vi "VI Tree.vi"   [LabVIEW 2018, in "Agilent N6700 Series.lvlib"]
doc: "This is the instrument driver for the Keysight/Agilent N6700 Series.\nThe VI Tree displays all the user-callable VIs of the instrument driver in an organized table."
uses:
  Agilent N6700 Series.lvlib
  Configuration/Waveform/Configure Waveform (Exponential).vi
  Configuration/Waveform/Sequence/Configure Sequence (Exponential).vi
panel:
  # "(c) 2004-2019  National Instruments.  ALL RIGHTS RESERVED."
  # "SEE DIAGRAM\nFOR VI TREE."
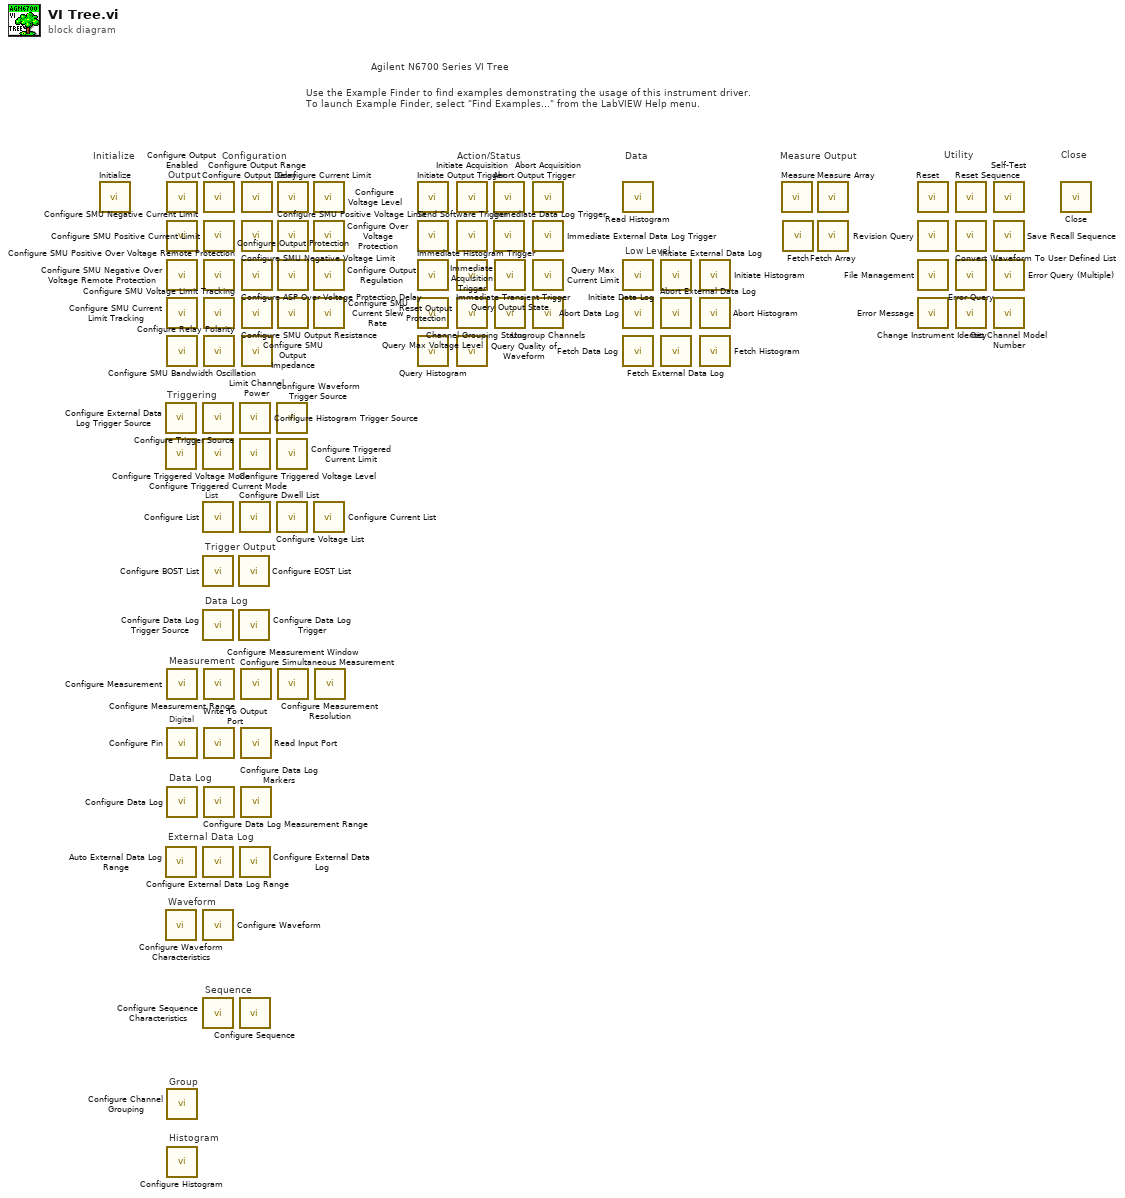
[diagram p0: block diagram]
diagram:
  # "External Data Log"
  # "Low Level"
  # "Sequence"
  # "Waveform"
  # "Data Log"
  # "Histogram"
  # "Data"
  # "Data Log"
  # "Measure Output"
  # "Agilent N6700 Series VI Tree"
  # "Use the Example Finder to find examples demonstrating the usage of this instrument driver.\nTo launch Example Finder, select \"Find Examples...\" from the LabVIEW Help menu."
  # "Configuration"
  # "Utility"
  # "Action/Status"
  # "Close"
  # "Initialize"
  # "Group"
  # "Digital"
  # "Measurement"
  # "Trigger Output"
  # "List"
  # "Triggering"
  # "Output"
  n1 = call "Initialize.vi"() -> ()  [unwired: 14 in, 2 out]
  n2 = call "Configure External Data Log Trigger Source.vi"() -> ()  [unwired: 10 in, 2 out]
  n3 = call "Configure Triggered Voltage Mode.vi"() -> ()  [unwired: 10 in, 2 out]
  n4 = call "Auto External Data Log Range.vi"() -> ()  [unwired: 10 in, 2 out]
  n5 = call "Configure Waveform Characteristics.vi"() -> ()  [unwired: 10 in, 2 out]
  n6 = call "Configure Output Enabled.vi"() -> ()  [unwired: 10 in, 2 out]
  n7 = call "Configure SMU Negative Current Limit.vi"() -> ()  [unwired: 10 in, 2 out]
  n8 = call "Configure SMU Negative Over Voltage Remote Protection.vi"() -> ()  [unwired: 10 in, 2 out]
  n9 = call "Configure SMU Current Limit Tracking.vi"() -> ()  [unwired: 10 in, 2 out]
  n10 = call "Configure SMU Bandwidth Oscillation.vi"() -> ()  [unwired: 10 in, 2 out]
  n11 = call "Configure Measurement.vi"() -> ()  [unwired: 10 in, 2 out]
  n12 = call "Configure Pin.vi"() -> ()  [unwired: 10 in, 2 out]
  n13 = call "Configure Data Log.vi"() -> ()  [unwired: 10 in, 2 out]
  n14 = call "Configure Channel Grouping.vi"() -> ()  [unwired: 10 in, 2 out]
  n15 = call "Configure Histogram.vi"() -> ()  [unwired: 10 in, 2 out]
  n16 = call "Configure Trigger Source.vi"() -> ()  [unwired: 10 in, 2 out]
  n17 = call "Configure Triggered Current Mode.vi"() -> ()  [unwired: 10 in, 2 out]
  n18 = call "Configure List.vi"() -> ()  [unwired: 10 in, 2 out]
  n19 = call "Configure BOST List.vi"() -> ()  [unwired: 10 in, 2 out]
  n20 = call "Configure Data Log Trigger Source.vi"() -> ()  [unwired: 10 in, 2 out]
  n21 = call "Configure External Data Log Range.vi"() -> ()  [unwired: 10 in, 2 out]
  n22 = call-poly "Configure Waveform.vi"() -> ()  [unwired: 14 in, 2 out]
  n23 = call "Configure Sequence Characteristics.vi"() -> ()  [unwired: 14 in, 2 out]
  n24 = call "Configure Output Delay.vi"() -> ()  [unwired: 10 in, 2 out]
  n25 = call "Configure SMU Positive Current Limit.vi"() -> ()  [unwired: 10 in, 2 out]
  n26 = call "Configure SMU Positive Over Voltage Remote Protection.vi"() -> ()  [unwired: 10 in, 2 out]
  n27 = call "Configure SMU Voltage Limit Tracking.vi"() -> ()  [unwired: 10 in, 2 out]
  n28 = call "Configure Relay Polarity.vi"() -> ()  [unwired: 10 in, 2 out]
  n29 = call "Configure Measurement Range.vi"() -> ()  [unwired: 10 in, 2 out]
  n30 = call "Write To Output Port.vi"() -> ()  [unwired: 10 in, 2 out]
  n31 = call "Configure Data Log Measurement Range.vi"() -> ()  [unwired: 10 in, 2 out]
  n32 = call "Configure EOST List.vi"() -> ()  [unwired: 10 in, 2 out]
  n33 = call "Configure Data Log Trigger.vi"() -> ()  [unwired: 10 in, 2 out]
  n34 = call "Configure Histogram Trigger Source.vi"() -> ()  [unwired: 10 in, 2 out]
  n35 = call "Configure Triggered Voltage Level.vi"() -> ()  [unwired: 10 in, 2 out]
  n36 = call "Configure Dwell List.vi"() -> ()  [unwired: 10 in, 2 out]
  n37 = call "Configure External Data Log.vi"() -> ()  [unwired: 10 in, 2 out]
  n38 = call-poly "Configure Sequence.vi"() -> ()  [unwired: 18 in, 2 out]
  n39 = call "Configure Simultaneous Measurement.vi"() -> ()  [unwired: 10 in, 2 out]
  n40 = call "Read Input Port.vi"() -> ()  [unwired: 9 in, 3 out]
  n41 = call "Configure Data Log Markers.vi"() -> ()  [unwired: 10 in, 2 out]
  n42 = call "Configure Output Range.vi"() -> ()  [unwired: 10 in, 2 out]
  n43 = call "Configure SMU Negative Voltage Limit.vi"() -> ()  [unwired: 10 in, 2 out]
  n44 = call "Configure ASP Over Voltage Protection Delay.vi"() -> ()  [unwired: 10 in, 2 out]
  n45 = call "Configure SMU Output Resistance.vi"() -> ()  [unwired: 10 in, 2 out]
  n46 = call "Limit Channel Power.vi"() -> ()  [unwired: 10 in, 2 out]
  n47 = call "Configure Waveform Trigger Source.vi"() -> ()  [unwired: 10 in, 2 out]
  n48 = call "Configure Triggered Current Limit.vi"() -> ()  [unwired: 10 in, 2 out]
  n49 = call "Configure Voltage List.vi"() -> ()  [unwired: 10 in, 2 out]
  n50 = call "Configure Current Limit.vi"() -> ()  [unwired: 10 in, 2 out]
  n51 = call "Configure SMU Positive Voltage Limit.vi"() -> ()  [unwired: 10 in, 2 out]
  n52 = call "Configure Output Protection.vi"() -> ()  [unwired: 10 in, 2 out]
  n53 = call "Configure SMU Output Impedance.vi"() -> ()  [unwired: 10 in, 2 out]
  n54 = call "Configure Measurement Window.vi"() -> ()  [unwired: 10 in, 2 out]
  n55 = call "Configure Voltage Level.vi"() -> ()  [unwired: 10 in, 2 out]
  n56 = call "Configure Over Voltage Protection.vi"() -> ()  [unwired: 10 in, 2 out]
  n57 = call "Configure Output Regulation.vi"() -> ()  [unwired: 14 in, 2 out]
  n58 = call "Configure SMU Current Slew Rate.vi"() -> ()  [unwired: 10 in, 2 out]
  n59 = call "Configure Current List.vi"() -> ()  [unwired: 10 in, 2 out]
  n60 = call "Configure Measurement Resolution.vi"() -> ()  [unwired: 10 in, 2 out]
  n61 = call "Initiate Output Trigger.vi"() -> ()  [unwired: 10 in, 2 out]
  n62 = call "Send Software Trigger.vi"() -> ()  [unwired: 10 in, 2 out]
  n63 = call "Immediate Histogram Trigger.vi"() -> ()  [unwired: 10 in, 2 out]
  n64 = call "Query Max Voltage Level.vi"() -> ()  [unwired: 9 in, 3 out]
  n65 = call "Query Histogram.vi"() -> ()  [unwired: 11 in, 5 out]
  n66 = call "Initiate Acquisition.vi"() -> ()  [unwired: 10 in, 2 out]
  n67 = call "Immediate Acquisition Trigger.vi"() -> ()  [unwired: 10 in, 2 out]
  n68 = call "Immediate Transient Trigger.vi"() -> ()  [unwired: 10 in, 2 out]
  n69 = call "Reset Output Protection.vi"() -> ()  [unwired: 10 in, 2 out]
  n70 = call "Query Quality of Waveform.vi"() -> ()  [unwired: 9 in, 3 out]
  n71 = call "Abort Output Trigger.vi"() -> ()  [unwired: 10 in, 2 out]
  n72 = call "Immediate Data Log Trigger.vi"() -> ()  [unwired: 10 in, 2 out]
  n73 = call "Query Output State.vi"() -> ()  [unwired: 9 in, 3 out]
  n74 = call "Channel Grouping Status.vi"() -> ()  [unwired: 9 in, 3 out]
  n75 = call "Abort Acquisition.vi"() -> ()  [unwired: 10 in, 2 out]
  n76 = call "Immediate External Data Log Trigger.vi"() -> ()  [unwired: 10 in, 2 out]
  n77 = call "Query Max Current Limit.vi"() -> ()  [unwired: 9 in, 3 out]
  n78 = call "Ungroup Channels.vi"() -> ()  [unwired: 10 in, 2 out]
  n79 = call "Read Histogram.vi"() -> ()  [unwired: 9 in, 3 out]
  n80 = call "Initiate Data Log.vi"() -> ()  [unwired: 10 in, 2 out]
  n81 = call "Abort Data Log.vi"() -> ()  [unwired: 10 in, 2 out]
  n82 = call "Fetch Data Log.vi"() -> ()  [unwired: 9 in, 3 out]
  n83 = call "Initiate External Data Log.vi"() -> ()  [unwired: 10 in, 2 out]
  n84 = call "Abort External Data Log.vi"() -> ()  [unwired: 10 in, 2 out]
  n85 = call "Fetch External Data Log.vi"() -> ()  [unwired: 9 in, 3 out]
  n86 = call "Initiate Histogram.vi"() -> ()  [unwired: 10 in, 2 out]
  n87 = call "Abort Histogram.vi"() -> ()  [unwired: 10 in, 2 out]
  n88 = call "Fetch Histogram.vi"() -> ()  [unwired: 9 in, 3 out]
  n89 = call "Measure.vi"() -> ()  [unwired: 9 in, 3 out]
  n90 = call "Fetch.vi"() -> ()  [unwired: 9 in, 3 out]
  n91 = call "Measure Array.vi"() -> ()  [unwired: 8 in, 4 out]
  n92 = call "Fetch Array.vi"() -> ()  [unwired: 8 in, 4 out]
  n93 = call "Reset.vi"() -> ()  [unwired: 14 in, 2 out]
  n94 = call "Revision Query.vi"() -> ()  [unwired: 12 in, 4 out]
  n95 = call "File Management.vi"() -> ()  [unwired: 10 in, 2 out]
  n96 = call "Error Message.vi"() -> ()  [unwired: 11 in, 5 out]
  n97 = call "Reset Sequence.vi"() -> ()  [unwired: 10 in, 2 out]
  n98 = call "Convert Waveform To User Defined List.vi"() -> ()  [unwired: 10 in, 2 out]
  n99 = call "Error Query.vi"() -> ()  [unwired: 12 in, 4 out]
  n100 = call "Change Instrument Identity.vi"() -> ()  [unwired: 10 in, 2 out]
  n101 = call "Self-Test.vi"() -> ()  [unwired: 12 in, 4 out]
  n102 = call "Save Recall Sequence.vi"() -> ()  [unwired: 10 in, 2 out]
  n103 = call "Error Query (Multiple).vi"() -> ()  [unwired: 12 in, 4 out]
  n104 = call "Get Channel Model Number.vi"() -> ()  [unwired: 9 in, 3 out]
  n105 = call "Close.vi"() -> ()  [unwired: 15 in, 1 out]
